vi "Run-Time Activation Checker.vi"() -> ()   [LabVIEW 2013]
uses:
  <vilib>/AddonLicensing/SoftwareKeyLicensingProvider.llb/_SK_LicenseFileInfo.ctl
  <vilib>/AddonLicensing/API.llb/_LV2P_ActivationInfo.ctl
  <vilib>/AddonLicensing/NI_LV2PLicAPI.lvlib
panel:
  out "valid license status?":bool
  out "license file path":path
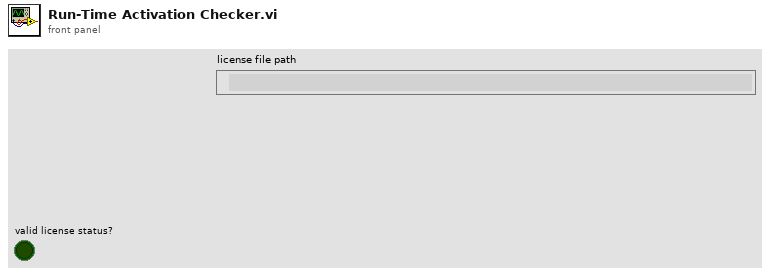
[diagram p1: front panel]
types:
  T1 = typedef "NI_LV2PLicAPI.lvlib/_LV2P_ActivationInfo.ctl" = cluster{"trigger code seed":i32, "encryption seed":i32, "activation server name":string, "activation server URL":string, "supports automatic activation":bool, "supports web activation":bool, "supports phone activation":bool, "web activation URL":string, "phone activation number":string, "purchase page URL":string}
  T2 = typedef "NI_LV2PLicAPI.lvlib/_SK_LicenseFileInfo.ctl" = cluster{"handle":i32, "full path":path, "password":string}
  T3 = enum16{"Invalid", "Expired", "Evaluation", "Activated"}
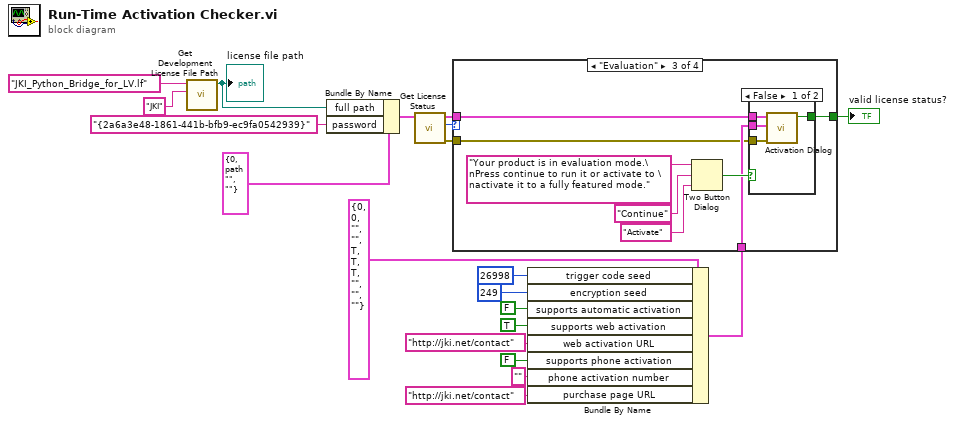
[diagram p0: block diagram]
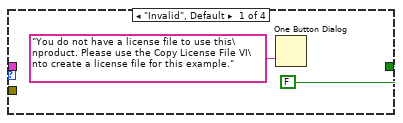
[diagram p2: hidden frame]
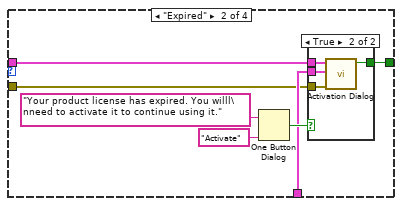
[diagram p3: hidden frame]
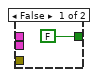
[diagram p4: hidden frame]
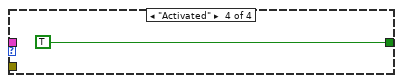
[diagram p6: hidden frame]
diagram:
  n1 = call <vilib>:"Get Development License File Path.vi"("company name"="JKI", "license file name"="JKI_Python_Bridge_for_LV.lf") -> ("license file path"=w17:path)  [unwired: 8 in, 1 out]
  "license file path" <- w17
  n2 = Bundle By Name(cluster=T2 {"handle"=0, "full path"=path "", "password"=""} ("license file info"), "full path"=w17, "password"="{2a6a3e48-1861-441b-bfb9-ec9fa0542939}") -> (w2:T2)
  n3 = call <vilib>:"Get License Status.vi"("license file info"=w2) -> ("error out"=w14:errorcluster, "license status"=w15:T3, "license file info out"=w13:T2)  [unwired: 7 in, 1 out]
  n4 = Bundle By Name(cluster=T1 {"trigger code seed"=0, "encryption seed"=0, "activation server name"="", "activation server URL"="", "supports automatic activation"=TRUE, "supports web activation"=TRUE, "supports phone activation"=TRUE, "web activation URL"="", "phone activation number"="", "purchase page URL"=""} ("activation info"), "trigger code seed"=26998, "encryption seed"=249 ("trigger code seed"), "supports automatic activation"=FALSE ("supports automated online"), "supports web activation"=TRUE ("supports web"), "web activation URL"="http://jki.net/contact" ("manual activation page"), "supports phone activation"=FALSE ("supports phone"), "phone activation number"="" ("phone number"), "purchase page URL"="http://jki.net/contact" ("product purchase page")) -> (w3:T1)
  n5 = case shown="\"Evaluation\"" w15 {
    tunnel: w14 -> [_ w24 w35 _]
    tunnel: w13 -> [_ w25 w37 _]
    tunnel: [FALSE ("activation successful?") w23 w38 TRUE] -> w12
    tunnel: w3 -> [_ w26 w36 _]
    frame "Invalid", Default {
      n6 = One Button Dialog(message="You do not have a license file to use this\nproduct. Please use the Copy License File VI\nto create a license file for this example.") -> ()  [unwired: 1 in, 1 out]
    }
    frame "Expired" {
      n7 = One Button Dialog(message="Your product license has expired. You willl\nneed to activate it to continue using it.", button name ("OK")="Activate") -> (true=w27:bool)
      n8 = case shown="True" w27 {
        tunnel: [FALSE ("activation successful?") w34] -> w23
        tunnel: w25 -> [_ w33]
        tunnel: w26 -> [_ w32]
        tunnel: w24 -> [_ w31]
        frame False {
        }
        frame True {
          n9 = call <vilib>:"Activation Dialog.vi"("error in (no error)"=w31, "activation info"=w32, "license file info"=w33) -> ("activation successful?"=w34:bool)  [unwired: 7 in, 1 out]
        }
      }
    }
    frame "Evaluation" {
      n10 = Two Button Dialog(message="Your product is in evaluation mode.\nPress continue to run it or activate to \nactivate it to a fully featured mode.", 1:"Activate" ("F button name (\"Cancel\")"), 2:"Continue" ("T button name (\"OK\")")) -> (T button?=w39:bool)
      n11 = case shown="False" w39 {
        selector: w39 -> [_ w47]
        tunnel: [w46 w47] -> w38
        tunnel: w37 -> [w45 _]
        tunnel: w36 -> [w44 _]
        tunnel: w35 -> [w43 _]
        frame False {
          n12 = call <vilib>:"Activation Dialog.vi"("error in (no error)"=w43, "activation info"=w44, "license file info"=w45) -> ("activation successful?"=w46:bool)  [unwired: 7 in, 1 out]
        }
        frame True {
        }
      }
    }
    frame "Activated" {
    }
  }
  "valid license status?" <- w12
